vi "Read TestCases.vi"(9 "TestSuite in":refnum<class "TestSuite.lvclass">) -> (3 "TestSuite out":refnum<class "TestSuite.lvclass">, 4 "TestCases":refnum<class "TestCase.lvclass">[](array[class]))   [LabVIEW 2014, in "TestSuite.lvclass"]
uses:
  TestSuite.lvclass
  TestCase/TestCase.lvclass
  TestSuite.lvclass/TestSuite.ctl
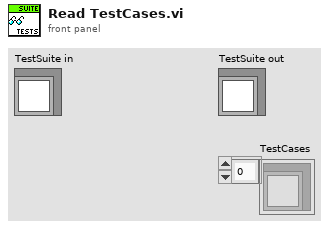
[diagram p1: front panel]
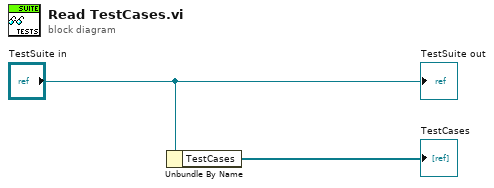
[diagram p0: block diagram]
diagram:
  n1 = Unbundle By Name("TestSuite in") -> ("TestCases"=→"TestCases":refnum<class "TestCase.lvclass">[])
  "TestSuite out" <- "TestSuite in"
